vi "Enumerate Cameras.vi"() -> (2 "Camera Info":T1(array[cluster]), 3 "Cameras":string[](array[string]))   [LabVIEW 2015]
uses:
  <vilib>/vision/driver/NI_Vision_Acquisition_Software.lvlib
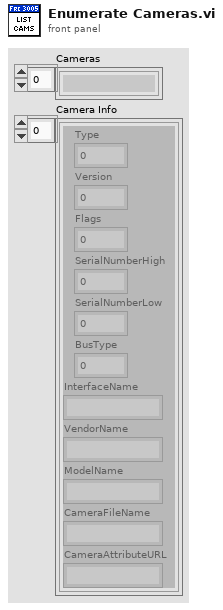
[diagram p1: front panel]
types:
  T1 = cluster{"Type":u32, "Version":u32, "Flags":u32, "SerialNumberHigh":u32, "SerialNumberLow":u32, "BusType":u32, "InterfaceName":string, "VendorName":string, "ModelName":string, "CameraFileName":string, "CameraAttributeURL":string}[]
  T2 = cluster{"Type":u32, "Version":u32, "Flags":u32, "SerialNumberHigh":u32, "SerialNumberLow":u32, "BusType":u32, "InterfaceName":string, "VendorName":string, "ModelName":string, "CameraFileName":string, "CameraAttributeURL":string}
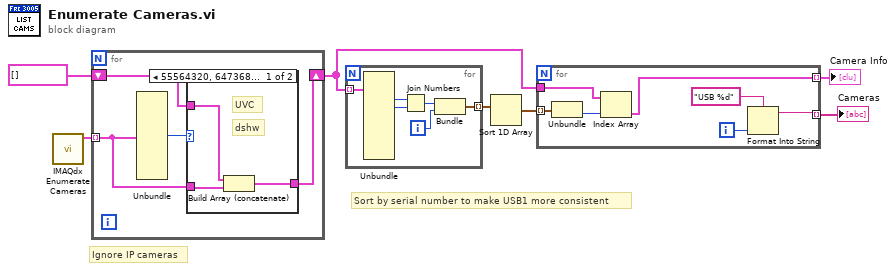
[diagram p0: block diagram]
diagram:
  # "Ignore IP cameras"
  # "Sort by serial number to make USB1 more consistent"
  n1 = call <vilib>:"IMAQdx Enumerate Cameras.vi"() -> ("Camera Information Array"=w7:T1)  [unwired: 10 in, 1 out]
  n2 = for {
    shift-right: [w8] -> w6
    shift-left: T1 [] -> [w9]
    tunnel: w7 -> [w10] mode=indexing
    n3 = Unbundle(w10) -> ("BusType"=w11:u32)  [unwired: 10 out]
    n4 = case shown="55564320, 64736877" w11 {
      tunnel: w10 -> [w13 _]
      tunnel: w9 -> [w14 w15]
      tunnel: [w12 w15] -> w8
      frame 1431716640, 1685284983 {
        # "dshw"
        # "UVC"
        n5 = Build Array (concatenate)(w14, w13) -> (w12:T1)
      }
      frame Default {
      }
    }
  }
  n6 = for {
    tunnel: w6 -> [w21] mode=indexing
    tunnel: [w16] -> w4 mode=indexing
    i -> [w17]
    n7 = Unbundle(w21) -> ("SerialNumberHigh"=w19:u32, "SerialNumberLow"=w20:u32)  [unwired: 9 out]
    n8 = Join Numbers(hi=w19, lo=w20) -> ((hi.lo)=w18:u64)
    n9 = Bundle(w18, w17) -> (w16:cluster{u64, i32})  [unwired: 1 in]
  }
  n10 = Sort 1D Array(array=w4) -> (sorted array=w5:cluster{u64, i32}[])
  n11 = for {
    tunnel: w5 -> [w28] mode=indexing
    tunnel: w6 -> [w26]
    tunnel: [w22] -> w2 mode=indexing
    tunnel: [w25] -> w1 mode=indexing
    i -> [w24]
    n12 = Unbundle(w28) -> (w27:i32)  [unwired: 1 out]
    n13 = Index Array(array=w26, index=w27) -> (element=w25:T2)
    n14 = Format Into String(format string="USB %d", w24) -> (resulting string=w22:string)  [unwired: 2 in, 1 out]
  }
  "Cameras" <- w2
  "Camera Info" <- w1
